vi "Rate Per Second.vi"(10 "Input Number":i32) -> (2 "Rate Per Second":i32)   [LabVIEW 2010]
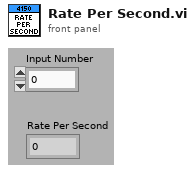
[diagram p1: front panel]
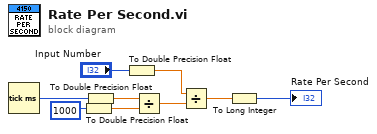
[diagram p0: block diagram]
diagram:
  n1 = Tick Count (ms)() -> (millisecond timer value=w8:u32)
  n2 = To Double Precision Float(number=1000) -> (double precision float=w3:dbl)
  n3 = To Double Precision Float(number=w8) -> (double precision float=w4:dbl)
  n4 = To Double Precision Float(number="Input Number") -> (double precision float=w5:dbl)
  n5 = Divide(x=w4, y=w3) -> (x/y=w9:dbl)
  n6 = Divide(x=w5, y=w9) -> (x/y=w2:dbl)
  n7 = To Long Integer(number=w2) -> (32bit integer=→"Rate Per Second":i32)
